vi "Practica_1y2_Punto_2_2.vi"() -> ()   [LabVIEW 2020]
uses:
  <vilib>/numeric/Random Number (Range) U64.vi
  <vilib>/numeric/sub_Random U32.vi
panel:
  out "min value":dbl
  out "max value":dbl
  out "Filtro EMA":dbl[](array[numeric])
  out "XY Graph":cluster{"Y":dbl[], "Y":dbl[]}[](graph)
  out "Grados Celsius":dbl[](array[numeric])
  out "Grados Farenheit":dbl[](array[numeric])
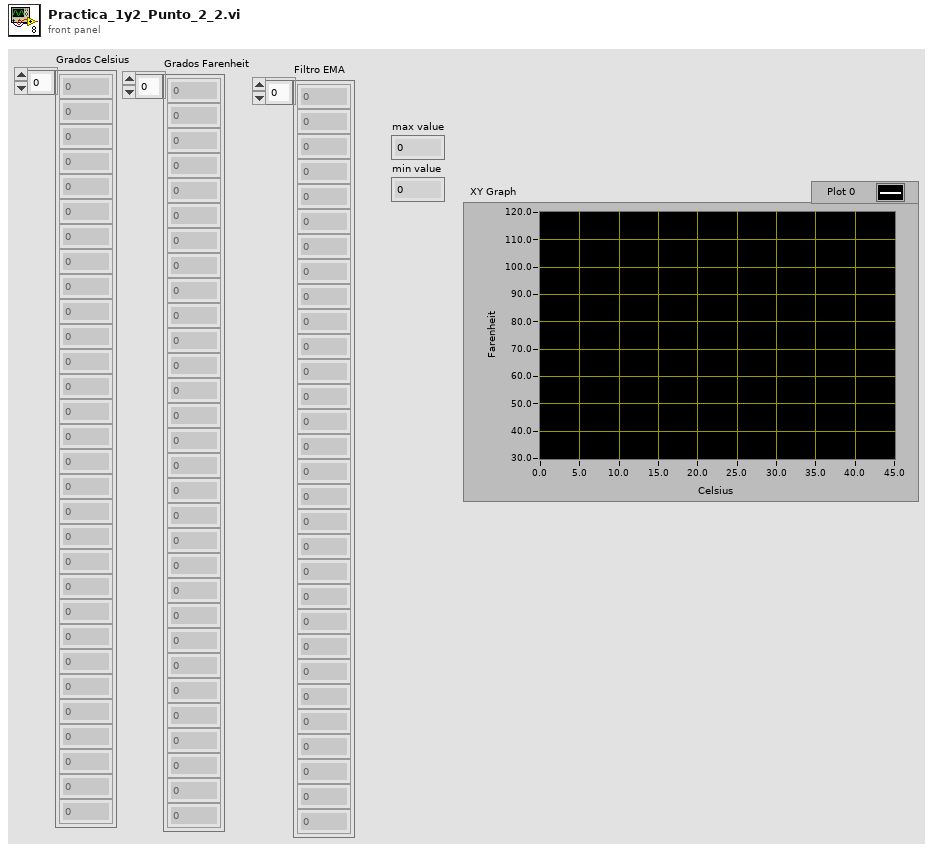
[diagram p1: front panel]
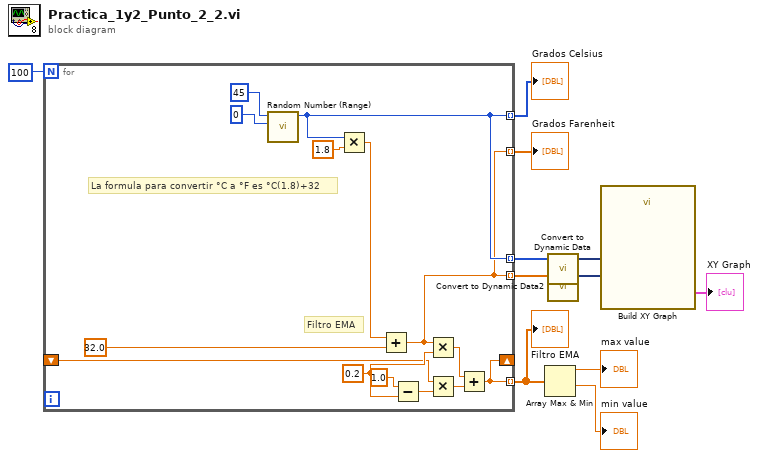
[diagram p0: block diagram]
diagram:
  n1 = for {
    N: 100 -> [_]
    tunnel: [w19] -> w10 mode=indexing
    tunnel: [w20] -> w9 mode=indexing
    tunnel: [w20] -> w7 mode=indexing
    tunnel: [w19] -> w5 mode=indexing
    shift-right: [w12] -> _
    shift-left: _ -> [w13]
    tunnel: [w12] -> w3 mode=indexing
    w16 = 0.2 ("y")
    # "Filtro EMA"
    # "La formula para convertir °C a °F es °C(1.8)+32"
    n2 = call-poly <vilib>:"Random Number (Range).vi"("lower bound (0)"=u64 0, "upper bound (100)"=u64 45) -> ("number"=w20:u64)  [unwired: 9 in]
    n3 = Multiply(x=w20, y=1.8) -> (x*y=w24:dbl)
    n4 = Add(x=w24, y=32.0) -> (x+y=w19:dbl)
    n5 = Subtract(x=1.0, y=w16) -> (x-y=w15:dbl)
    n6 = Multiply(x=w19, y=w16) -> (x*y=w18:dbl)
    n7 = Multiply(x=w13, y=w15) -> (x*y=w14:dbl)
    n8 = Add(x=w18, y=w14) -> (x+y=w12:dbl)
  }
  "Grados Farenheit" <- w10
  "Grados Celsius" <- w9
  "Filtro EMA" <- w3
  n9 = Array Max & Min(array=w3) -> (max value=→"max value":dbl, min value=→"min value":dbl)  [unwired: 2 out]
  n10 = call "Convert to Dynamic Data"("Array"=w7) -> ("Dynamic Data Type"=w6:dynamicdata)  [unwired: 3 in]
  n11 = call "Convert to Dynamic Data2"("Array"=w5) -> ("Dynamic Data Type"=w4:dynamicdata)  [unwired: 3 in]
  n12 = call "Build XY Graph"("Y Input"=w4, "X Input"=w6) -> ("XY Graph"=→"XY Graph":cluster{"X":dbl[], "Y":dbl[]}[])  [unwired: 8 in, 1 out]
